vi "Avg Done.vi"(8 "error in (no error)":errorcluster, 10 "Avg Done":bool, 11 "Controller in":refnum<class "Controller.lvclass">) -> (0 "error out":errorcluster, 3 "Controller out":refnum<class "Controller.lvclass">)   [LabVIEW 2022 SP3, in "Controller.lvlib" / "Controller.lvclass"]
uses:
  Controller.lvclass
  Controller.lvclass/Controller.ctl
  UserInterface/UserInterface Messages/Log Data Msg/Log Data Msg.lvclass
  ImageHandler/ImageHandler Messages/Init Msg/Init Msg.lvclass
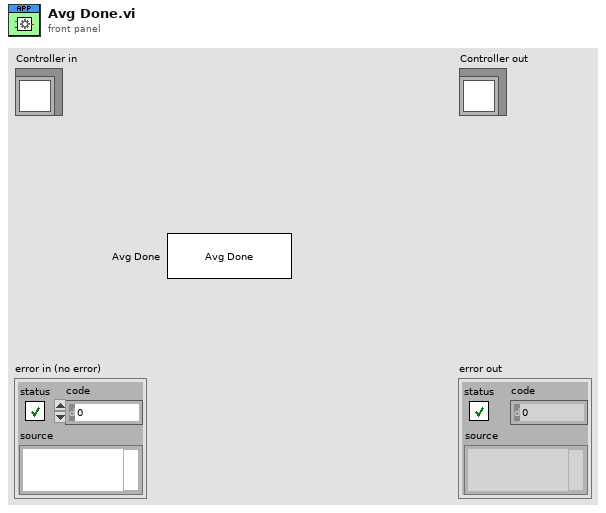
[diagram p1: front panel]
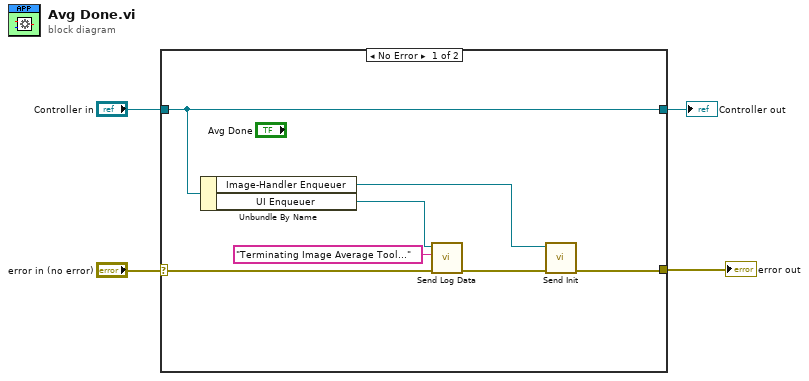
[diagram p0: block diagram]
diagram:
  n1 = case shown="No Error" "error in (no error)" {
    selector: "error in (no error)" -> [w11 w12]
    tunnel: "Controller in" -> [w5 w13]
    tunnel: [w7 w12] -> w3
    tunnel: [w5 w13] -> w1
    frame No Error {
      n2 = Unbundle By Name(w5) -> ("Image-Handler Enqueuer"=w6:refnum<class "Message Enqueuer.lvclass">, "UI Enqueuer"=w9:refnum<class "Message Enqueuer.lvclass">)
      n3 = call "Send Log Data.vi"("error in (no error)"=w11, "Message"="Terminating Image Average Tool...", "Message Enqueuer"=w9) -> ("error out"=w10:errorcluster)  [unwired: 7 in, 1 out]
      n4 = call "Send Init.vi"("error in (no error)"=w10, "Message Enqueuer"=w6) -> ("error out"=w7:errorcluster)  [unwired: 8 in, 1 out]
    }
    frame Error {
    }
  }
  "error out" <- w3
  "Controller out" <- w1
